vi "LTVDiffDriveCtrl_AtReference.vi"(11 "LTV_DIFF_DRIVE_CTRL":T1) -> (3 "At Reference":bool)   [LabVIEW 2019, in "Trajectory_Library.lvlib"]
doc: "Create implicit model follower\n\nInputs:\n - A < states, states > -- Continuous system matrix of the plant being controlled.\n - B < states, inputs > -- Continuous input matrix of the plant being controlled.\n - A_Ref < states, states > -- Continuous system matrix whose dymanics should be followed.\n - B_Ref < states, inputs > -- Continuous input matrix x whose dymanics should be followed.\n\nOutputs:\n - Error -- If TRUE, an error occured."
uses:
  <vilib>/Analysis/Matrix/Datatypes/RealMatrix.ctl
  Trajectory_Library.lvlib
  <vilib>/Analysis/Matrix/NI_Matrix.lvlib
  FUNCTION_GENERATOR_MATRIX.ctl
  LTV_DIFF_DRIVE_CTRL.ctl
panel:
  # "< 5, 1 >"
  # "< 5, 1 >"
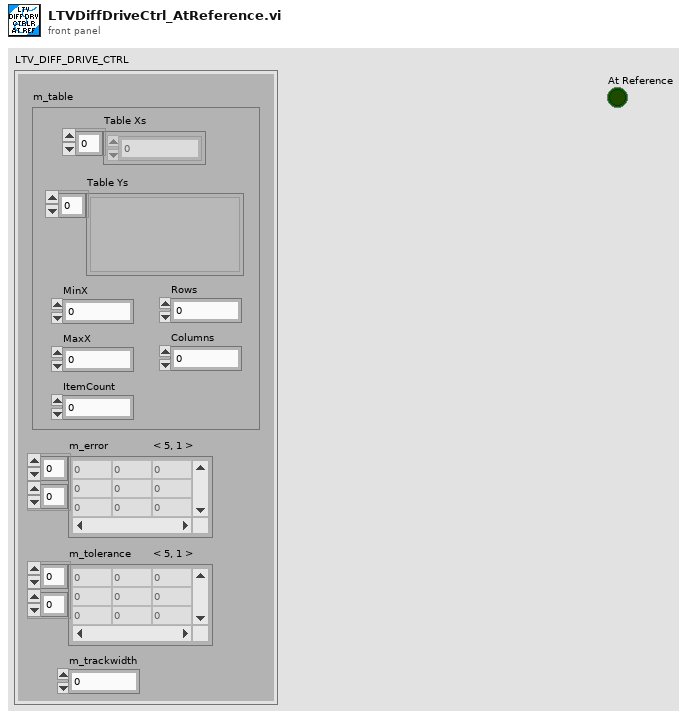
[diagram p1: front panel]
types:
  T1 = typedef "Trajectory_Library.lvlib/LTV_DIFF_DRIVE_CTRL.ctl" = cluster{"m_table":T2, "m_error":T3, "m_tolerance":T3, "m_trackwidth":dbl}
  T2 = typedef "Trajectory_Library.lvlib/FUNCTION_GENERATOR_MATRIX.ctl" = cluster{"Table Xs":dbl[], "Table Ys":variant[], "MinX":dbl, "MaxX":dbl, "ItemCount":i32, "Rows":i32, "Columns":i32}
  T3 = typedef "NI_Matrix.lvlib/RealMatrix.ctl" = dbl[][]
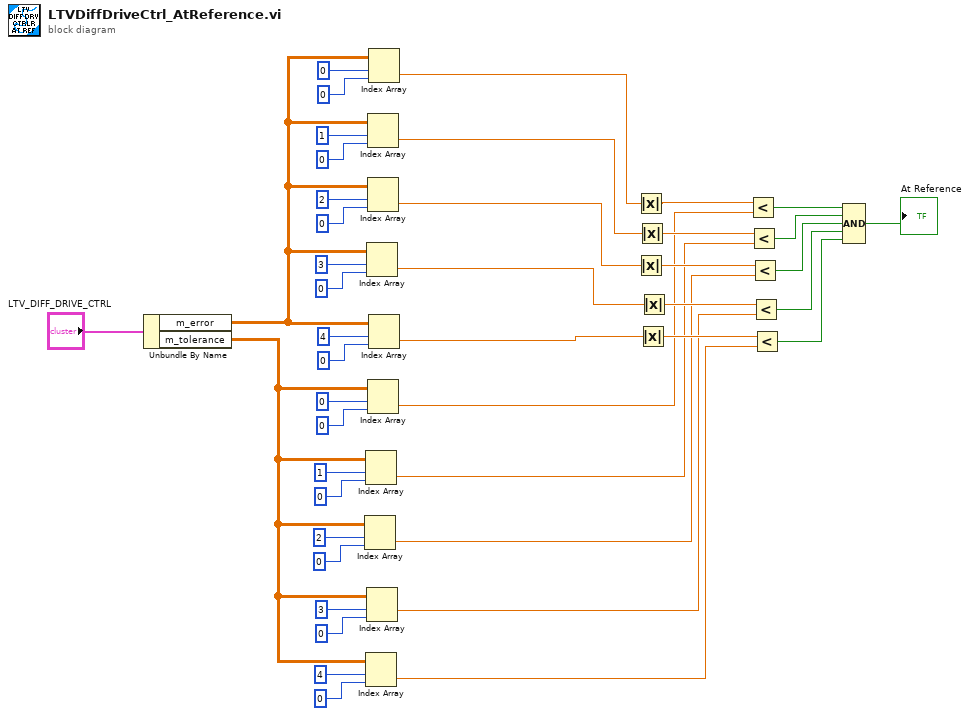
[diagram p0: block diagram]
diagram:
  n1 = Unbundle By Name("LTV_DIFF_DRIVE_CTRL") -> ("m_error"=w11:T3, "m_tolerance"=w12:T3)
  n2 = Index Array(array=w12, index (row)=2, index (col)=0) -> (element=w3:dbl)
  n3 = Index Array(array=w12, index (row)=1, index (col)=0) -> (element=w4:dbl)
  n4 = Index Array(array=w12, index (row)=4, index (col)=0) -> (element=w1:dbl)
  n5 = Index Array(array=w11, index (row)=3, index (col)=0) -> (element=w7:dbl)
  n6 = Index Array(array=w12, index (row)=3, index (col)=0) -> (element=w2:dbl)
  n7 = Index Array(array=w11, index (row)=1, index (col)=0) -> (element=w9:dbl)
  n8 = Index Array(array=w11, index (row)=2, index (col)=0) -> (element=w8:dbl)
  n9 = Index Array(array=w12, index (row)=0, index (col)=0) -> (element=w5:dbl)
  n10 = Index Array(array=w11, index (row)=0, index (col)=0) -> (element=w10:dbl)
  n11 = Index Array(array=w11, index (row)=4, index (col)=0) -> (element=w6:dbl)
  n12 = Absolute Value(x=w10) -> (abs(x)=w43:dbl)
  n13 = Absolute Value(x=w8) -> (abs(x)=w41:dbl)
  n14 = Absolute Value(x=w9) -> (abs(x)=w42:dbl)
  n15 = Absolute Value(x=w6) -> (abs(x)=w35:dbl)
  n16 = Absolute Value(x=w7) -> (abs(x)=w36:dbl)
  n17 = Less?(x=w43, y=w5) -> (x < y?=w40:bool)
  n18 = Less?(x=w42, y=w4) -> (x < y?=w39:bool)
  n19 = Less?(x=w41, y=w3) -> (x < y?=w38:bool)
  n20 = Less?(x=w36, y=w2) -> (x < y?=w34:bool)
  n21 = Less?(x=w35, y=w1) -> (x < y?=w33:bool)
  n22 = Compound Arithmetic op=AND(w40, w39, w38, w34, w33) -> (→"At Reference":bool)
